vi "_script_fix_Parse State Queue in Find Parse State Queue vi name2.vi"   [LabVIEW 2014]
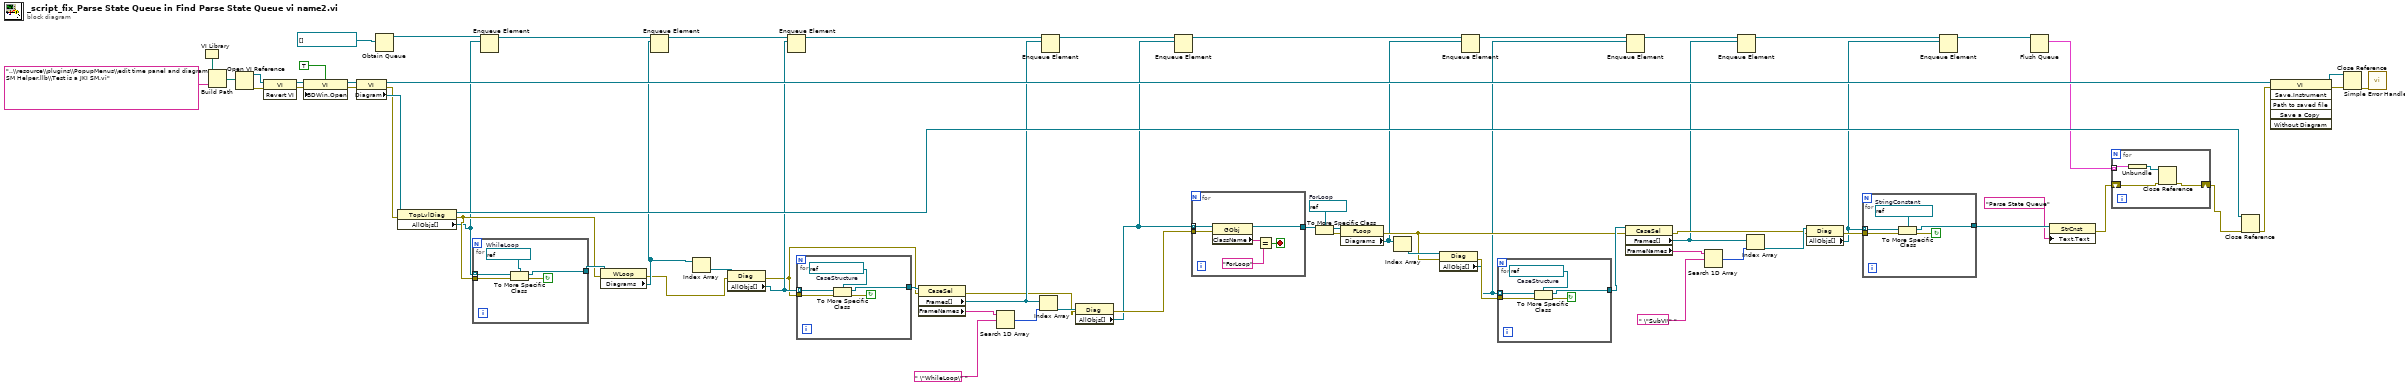
[diagram p0: block diagram]
diagram:
  w57 = refnum<vi> refnum  # ForLoop
  n1 = VI Library() -> (path=w67:path)
  n2 = Build Path(base path=w67, name or relative path="..\\resource\\plugins\\PopupMenus\\edit time panel and diagram\\JKI SM Helper.llb\\Test is a JKI SM.vi") -> (appended path=w65:path)
  n3 = Open VI Reference(vi path=w65) -> (vi reference=w68:refnum<vi>, error out=w69:errorcluster)  [unwired: 5 in]
  n4 = invoke class="VI" method="Revert VI"(reference=w68, error in=w69) -> (reference out=w49:refnum<vi>, error out=w48:errorcluster)  [unwired: 1 in, 1 out]
  n5 = property class="VI"(reference=w49, error in=w48, "BDWin.Open"=TRUE ("Block Diagram Window:Open")) -> (reference out=w47:refnum<vi>, error out=w46:errorcluster)
  n6 = property class="VI"(reference=w47, error in=w46) -> (reference out=w64:refnum<vi>, error out=w59:errorcluster, "Diagram"=w60:refnum<vi>)
  n7 = Obtain Queue(element data type=refnum<vi>[] [] ("All Objects[]")) -> (queue out=w32:refnum<queue>)  [unwired: 4 in, 2 out]
  n8 = property class="TopLvlDiag"(reference=w60, error in=w59) -> (reference out=w51:refnum<vi>, error out=w34:errorcluster, "AllObjs[]"=w31:refnum<vi>[])
  n9 = for {
    tunnel: w31 -> [w74] mode=indexing
    tunnel: w34 -> [w73]
    tunnel: [w71] -> w35
    stop <- w72 continue-if-true
    w70 = refnum<vi> refnum  # WhileLoop
    n10 = To More Specific Class(target class=w70, reference=w74, error in=w73) -> (specific class reference=w71:refnum<vi>, error out=w72:errorcluster)
  }
  n11 = Enqueue Element(queue=w32, element=w31) -> (queue out=w30:refnum<queue>)  [unwired: 2 in, 2 out]
  n12 = property class="WLoop"(reference=w35, error in=w34) -> (error out=w27:errorcluster, "Diagrams"=w29:refnum<vi>[])  [unwired: 1 out]
  n13 = Enqueue Element(queue=w30, element=w29) -> (queue out=w25:refnum<queue>)  [unwired: 2 in, 2 out]
  n14 = Index Array(array=w29) -> (element=w28:refnum<vi>)  [unwired: 1 in]
  n15 = property class="Diag"(reference=w28, error in=w27) -> (error out=w18:errorcluster, "AllObjs[]"=w26:refnum<vi>[])  [unwired: 1 out]
  n16 = Enqueue Element(queue=w25, element=w26) -> (queue out=w20:refnum<queue>)  [unwired: 2 in, 2 out]
  n17 = for {
    tunnel: w26 -> [w79] mode=indexing
    tunnel: w18 -> [w78]
    tunnel: [w76] -> w21
    stop <- w77 continue-if-true
    w75 = refnum<vi> refnum  # CaseStructure
    n18 = To More Specific Class(target class=w75, reference=w79, error in=w78) -> (specific class reference=w76:refnum<vi>, error out=w77:errorcluster)
  }
  n19 = property class="CaseSel"(reference=w21, error in=w18) -> (error out=w16:errorcluster, "Frames[]"=w19:refnum<vi>[], "FrameNames"=w22:string[])  [unwired: 1 out]
  n20 = Search 1D Array(1D array=w22, element=" \"WhileLoop\" " ("y")) -> (index of element=w24:i32)  [unwired: 1 in]
  n21 = Index Array(array=w19, index=w24) -> (element=w17:refnum<vi>)
  n22 = Enqueue Element(queue=w20, element=w19) -> (queue out=w13:refnum<queue>)  [unwired: 2 in, 2 out]
  n23 = property class="Diag"(reference=w17, error in=w16) -> (error out=w15:errorcluster, "AllObjs[]"=w14:refnum<vi>[])  [unwired: 1 out]
  n24 = Enqueue Element(queue=w13, element=w14) -> (queue out=w11:refnum<queue>)  [unwired: 2 in, 2 out]
  n25 = for {
    tunnel: w14 -> [w85] mode=indexing
    tunnel: w15 -> [w84]
    tunnel: [w83] -> w58
    stop <- w80 stop-if-true
    n26 = property class="GObj"(reference=w85, error in=w84) -> (reference out=w83:refnum<vi>, "ClassName"=w82:string)  [unwired: 1 out]
    n27 = Equal?(x=w82, y="ForLoop") -> (x = y?=w80:bool)
  }
  n28 = To More Specific Class(target class=w57, reference=w58) -> (specific class reference=w56:refnum<vi>, error out=w55:errorcluster)  [unwired: 1 in]
  n29 = property class="FLoop"(reference=w56, error in=w55) -> (error out=w41:errorcluster, "Diagrams"=w12:refnum<vi>[])  [unwired: 1 out]
  n30 = Index Array(array=w12) -> (element=w44:refnum<vi>)  [unwired: 1 in]
  n31 = property class="Diag"(reference=w44, error in=w41) -> (error out=w43:errorcluster, "AllObjs[]"=w9:refnum<vi>[])  [unwired: 1 out]
  n32 = Enqueue Element(queue=w11, element=w12) -> (queue out=w10:refnum<queue>)  [unwired: 2 in, 2 out]
  n33 = for {
    tunnel: w9 -> [w90] mode=indexing
    tunnel: w43 -> [w89]
    tunnel: [w87] -> w42
    stop <- w88 continue-if-true
    w86 = refnum<vi> refnum  # CaseStructure
    n34 = To More Specific Class(target class=w86, reference=w90, error in=w89) -> (specific class reference=w87:refnum<vi>, error out=w88:errorcluster)
  }
  n35 = property class="CaseSel"(reference=w42, error in=w41) -> (error out=w36:errorcluster, "Frames[]"=w8:refnum<vi>[], "FrameNames"=w40:string[])  [unwired: 1 out]
  n36 = Enqueue Element(queue=w10, element=w9) -> (queue out=w7:refnum<queue>)  [unwired: 2 in, 2 out]
  n37 = Search 1D Array(1D array=w40, element=" \"SubVI\" " ("y")) -> (index of element=w38:i32)  [unwired: 1 in]
  n38 = Enqueue Element(queue=w7, element=w8) -> (queue out=w6:refnum<queue>)  [unwired: 2 in, 2 out]
  n39 = Index Array(array=w8, index=w38) -> (element=w37:refnum<vi>)
  n40 = property class="Diag"(reference=w37, error in=w36) -> (error out=w54:errorcluster, "AllObjs[]"=w5:refnum<vi>[])  [unwired: 1 out]
  n41 = for {
    tunnel: w5 -> [w95] mode=indexing
    tunnel: w54 -> [w94]
    tunnel: [w91] -> w53
    stop <- w92 continue-if-true
    w93 = refnum<vi> refnum  # StringConstant
    n42 = To More Specific Class(target class=w93, reference=w95, error in=w94) -> (specific class reference=w91:refnum<vi>, error out=w92:errorcluster)
  }
  n43 = Enqueue Element(queue=w6, element=w5) -> (queue out=w4:refnum<queue>)  [unwired: 2 in, 2 out]
  n44 = Flush Queue(queue=w4) -> (remaining elements=w3:cluster{"All Objects[]":refnum<vi>[]}[])  [unwired: 1 in, 2 out]
  n45 = property class="StrCnst"(reference=w53, "Text.Text"="Parse State Queue") -> (error out=w2:errorcluster)  [unwired: 1 in, 1 out]
  n46 = for {
    tunnel: w3 -> [w99] mode=indexing
    shift-right: [w96] -> w1
    shift-left: w2 -> [w97]
    n47 = Unbundle(w99) -> ("All Objects[]"=w98:refnum<vi>[])
    n48 = Close Reference(reference=w98, error in (no error)=w97) -> (error out=w96:errorcluster)
  }
  n49 = Close Reference(reference=w51, error in (no error)=w1) -> (error out=w50:errorcluster)
  n50 = invoke class="VI" method="Save.Instrument"(reference=w64, error in=w50) -> (reference out=w62:refnum<vi>, error out=w63:errorcluster)  [unwired: 4 in, 4 out]
  n51 = Close Reference(reference=w62, error in (no error)=w63) -> (error out=w61:errorcluster)
  n52 = call <vilib>:"Simple Error Handler.vi"("error in (no error)"=w61) -> ()  [unwired: 4 in, 5 out]
